vi "GetgitRevision.vi"(11 "File Path Control":path caption="File Path Control (leave blank to use Constants_Global value of EnFlo SW Folder)") -> (0 "status&log error":string, 1 "LocalModifications":string, 2 "branch":string, 3 "OverallRevision":string)   [LabVIEW 2022 SP3]
doc: "This VI uses the system's installed svn (subversion) software to return the revision number of the selected folder. Leaving the selected folder blank will use the global value of \"EnFlo SW Folder\".\nThe \"Overall Revision\" is the highest revision number in the entire hierarchy, recursing upwards as well as downwards- in other words, the revision which was checked out. The \"This Folder\" data is specific to the last changes to the selected folder."
uses:
  <vilib>/Utility/error.llb/Trim Whitespace One-Sided.vi
  Globals/Constants_global.vi
  <vilib>/regexp/Match Regular Expression.xnode
panel:
  out "This Folder's Last Changed Date":string
  out "This Folder Last Committed By":string
  out "status&log output":string
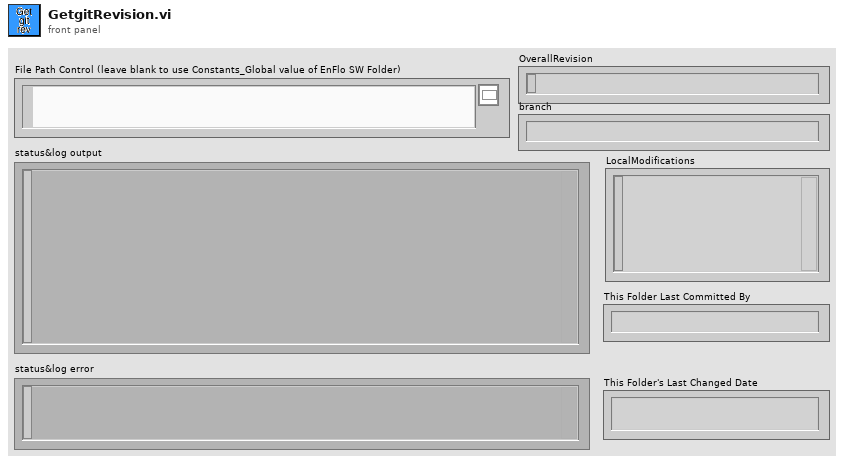
[diagram p1: front panel]
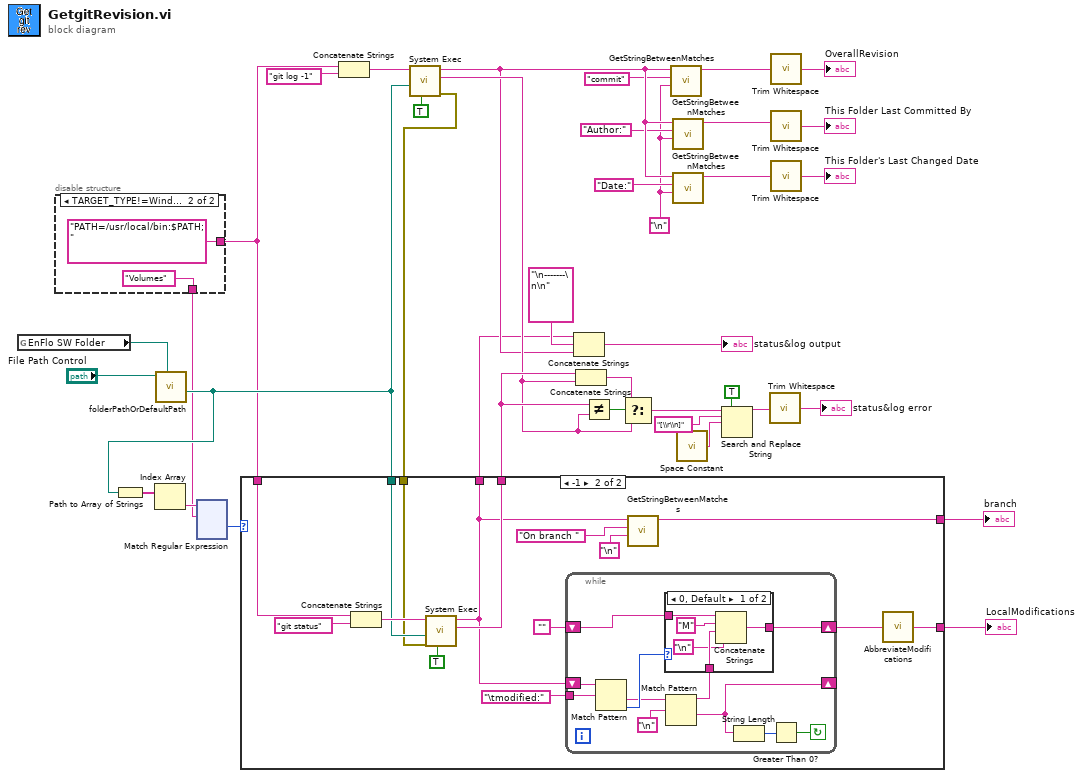
[diagram p0: block diagram]
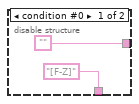
[diagram p2: hidden frame]
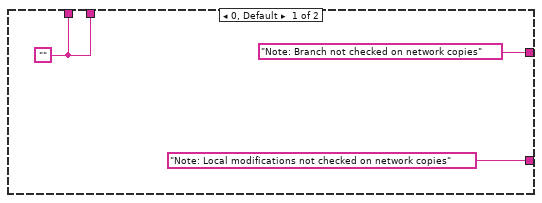
[diagram p3: hidden frame]
diagram:
  w11 = "\n" ("regular expression")
  n1 = global read "Constants_global.vi" "EnFlo SW Folder"() -> (w20:path)
  n2 = disable-structure shown="TARGET_TYPE!=Windows" {
    disable-tunnel: ["" ("command line") "PATH=/usr/local/bin:$PATH; " ("command line")] -> w2
    disable-tunnel: ["[F-Z]" ("regular expression") "Volumes" ("regular expression")] -> w3
    frame condition #0 {
    }
    frame condition #1 (active) {
    }
  }
  n3 = call "folderPathOrDefaultPath.vi"("defaultPath"=w20, "File Path Control"="File Path Control") -> ("folder"=w4:path)  [unwired: 8 in, 1 out]
  n4 = Path to Array of Strings(0:w4) -> (2:w7:string[])  [unwired: 1 out]
  n5 = Index Array(array=w7) -> (element=w6:string)  [unwired: 1 in]
  n6 = xnode "Match Regular Expression"("input string"=w6, "regular expression"=w3) -> ("offset past match"=w5:i32)  [unwired: 4 in, 4 out]
  n7 = Concatenate Strings(w2, "git log -1" ("command line")) -> (w26:string)
  n8 = call <vilib>:"System Exec.vi"("run minimized? (F)"=TRUE, "working directory"=w4, "command line"=w26) -> ("error out"=w8:errorcluster, "standard error"=w32:string, "standard output"=w17:string)  [unwired: 5 in, 1 out]
  n9 = case shown="-1" w5 {
    tunnel: [w45 w60] -> w35
    tunnel: w2 -> [_ w57]
    tunnel: w4 -> [_ w54]
    tunnel: [w45 w52] -> w10
    tunnel: ["Note: Branch not checked on network copies" ("VInames") w49] -> w9
    tunnel: ["Note: Local modifications not checked on network copies" ("VInames") w47] -> w1
    tunnel: w8 -> [_ w46]
    frame 0, Default {
      w45 = ""
    }
    frame -1 {
      n10 = Concatenate Strings(w57, "git status" ("command line")) -> (w59:string)
      n11 = call <vilib>:"System Exec.vi"("run minimized? (F)"=TRUE, "error in (no error)"=w46, "working directory"=w54, "command line"=w59) -> ("standard error"=w60:string, "standard output"=w52:string)  [unwired: 4 in, 2 out]
      n12 = while {
        shift-right: [w62] -> _
        shift-left: w52 -> [w71]
        shift-right: [w69] -> w48
        shift-left: "" -> [w68]
        tunnel: "\tmodified:" ("search string/char (-)") -> [w70]
        stop <- w66 continue-if-true
        n13 = Match Pattern(string=w71, regular expression=w70) -> (after substring=w63:string, offset past match=w65:i32)  [unwired: 1 in, 2 out]
        n14 = Match Pattern(string=w63, regular expression="\n") -> (before substring=w64:string, after substring=w62:string)  [unwired: 1 in, 2 out]
        n15 = case shown="0, Default" w65 {
          tunnel: [w76 w77] -> w69
          tunnel: w68 -> [w75 w77]
          tunnel: w64 -> [w73 _]
          frame 0, Default {
            n16 = Concatenate Strings(w75, "M" ("string"), w73, "\n") -> (w76:string)
          }
          frame -1 {
          }
        }
        n17 = String Length(string=w62) -> (length=w67:i32)
        n18 = Greater Than 0?(x=w67) -> (x > 0?=w66:bool)
      }
      n19 = call "GetStringBetweenMatches.vi"("postTarget"="\n" ("regular expression"), "preTarget"="On branch ", "stringIn"=w52) -> ("target"=w49:string)  [unwired: 7 in, 1 out]
      n20 = call "AbbreviateModifications.vi"("svnString"=w48) -> ("VInames"=w47:string)  [unwired: 4 in]
    }
  }
  "LocalModifications" <- w1
  "branch" <- w9
  n21 = Concatenate Strings(w10, "\n-------\n\n" ("string"), w17) -> (→"status&log output":string)
  n22 = Concatenate Strings(w35, w32) -> (w33:string)
  n23 = Not Equal?(x=w35, y=w32) -> (x != y?=w34:bool)
  n24 = Select(t=w33, s=w34, f=w32) -> (s? t:f=w28:string)
  n25 = call "GetStringBetweenMatches.vi"("postTarget"=w11, "preTarget"="commit" ("regular expression"), "stringIn"=w17) -> ("target"=w18:string)  [unwired: 7 in, 1 out]
  n26 = call "GetStringBetweenMatches.vi"("postTarget"=w11, "preTarget"="Author:" ("regular expression"), "stringIn"=w17) -> ("target"=w13:string)  [unwired: 7 in, 1 out]
  n27 = call "GetStringBetweenMatches.vi"("postTarget"=w11, "preTarget"="Date:" ("regular expression"), "stringIn"=w17) -> ("target"=w12:string)  [unwired: 7 in, 1 out]
  n28 = call <vilib>:"Space Constant.vi"() -> ("String"=w30:string)
  n29 = Search and Replace String(replace all?=TRUE ("replace all? (F)"), input string=w28, search string="[\\r\\n]", replace string=w30) -> (result string=w27:string)  [unwired: 4 in, 3 out]
  n30 = call <vilib>:"Trim Whitespace.vi"("string"=w27) -> ("trimmed string"=→"status&log error":string)  [unwired: 1 in]
  n31 = call <vilib>:"Trim Whitespace.vi"("string"=w18) -> ("trimmed string"=→"OverallRevision":string)  [unwired: 1 in]
  n32 = call <vilib>:"Trim Whitespace.vi"("string"=w13) -> ("trimmed string"=→"This Folder Last Committed By":string)  [unwired: 1 in]
  n33 = call <vilib>:"Trim Whitespace.vi"("string"=w12) -> ("trimmed string"=→"This Folder's Last Changed Date":string)  [unwired: 1 in]
